vi "Virtual traverse profile.vi"(6 "N_pts":i32=100, 8 "P_end":sgl[](array[numeric])=[10.0, 0.0, 0.0], 9 "P_start":sgl[](array[numeric])=[0.0, 0.0, 0.0], 10 "U_inf":sgl[](array[numeric])=[1.0, 0.0, 0.0], 11 "Panel triangles in":T1[](array[typedef])) -> (0 "V":sgl[](array[numeric]), 1 "U":sgl[](array[numeric]), 2 "z":sgl[](array[numeric]), 3 "y":sgl[](array[numeric]), 4 "W":sgl[](array[numeric]), 5 "x":sgl[](array[numeric]))   [LabVIEW 2017]
uses:
  ctls/Triangle panel.ctl
panel:
  # "PN 26/10/17"
  # "Vertices"
  # "Edges"
  # "Unit normal"
  # "Control point"
  # "Edge\nlinks \n(tri index)"
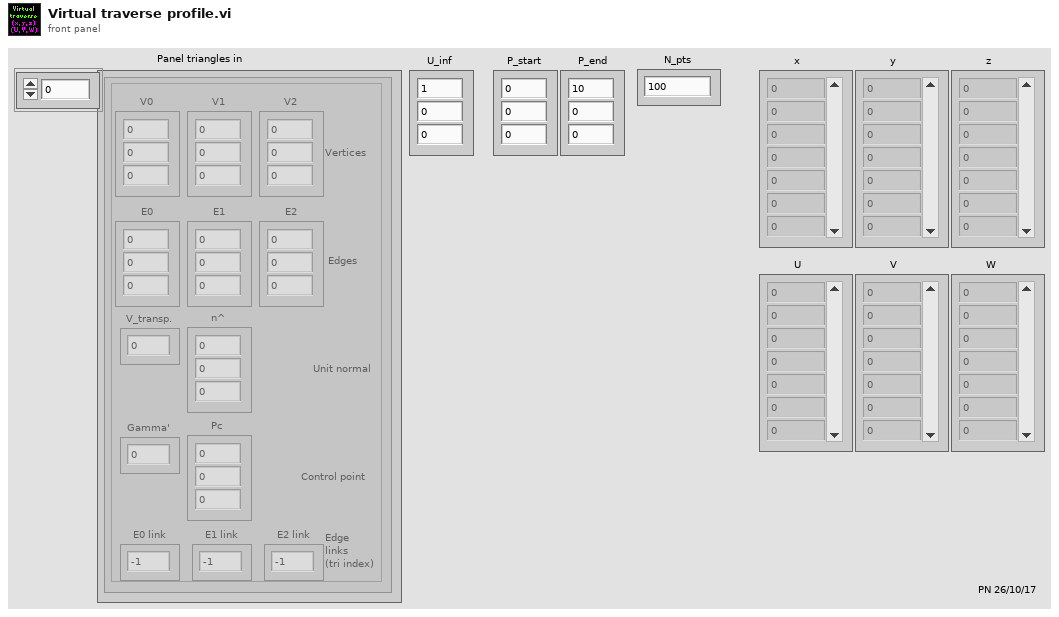
[diagram p1: front panel]
types:
  T1 = typedef "Triangle panel.ctl" = cluster{"V0":sgl[], "V1":sgl[], "V2":sgl[], "E0":sgl[], "E1":sgl[], "E2":sgl[], "n^":sgl[], "Pc":sgl[], "Gamma'":sgl, "V_transp.":sgl, "E0 link":i32, "E1 link":i32, "E2 link":i32}
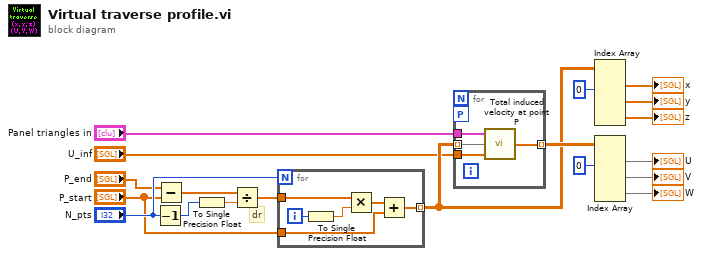
[diagram p0: block diagram]
diagram:
  # "dr"
  n1 = Decrement(x="N_pts") -> (x-1=w17:i32)
  n2 = Subtract(x="P_end", y="P_start") -> (x-y=w19:sgl[])
  n3 = To Single Precision Float(number=w17) -> (single precision float=w18:sgl)
  n4 = Divide(x=w19, y=w18) -> (x/y=w15:sgl[])
  n5 = for {
    N: "N_pts" -> [_]
    tunnel: "P_start" -> [w22]
    tunnel: w15 -> [w23]
    tunnel: [w20] -> w13 mode=indexing
    i -> [w25]
    n6 = To Single Precision Float(number=w25) -> (single precision float=w24:sgl)
    n7 = Multiply(x=w23, y=w24) -> (x*y=w21:sgl[])
    n8 = Add(x=w21, y=w22) -> (x+y=w20:sgl[])
  }
  n9 = for {
    tunnel: w13 -> [w28] mode=indexing
    tunnel: "Panel triangles in" -> [w29]
    tunnel: [w26] -> w14 mode=indexing
    tunnel: "U_inf" -> [w27]
    workers-P: _ -> [_]
    n10 = call "Total induced velocity at point P.vi"("U_inf"=w27, "P"=w28, "Triangle panels"=w29) -> ("(U, V, W) at P"=w26:sgl[])
  }
  n11 = Index Array(array=w13, index (col) #1=0 ("disabled index (col)")) -> (element #1=→"x":sgl[], element #2=→"y":sgl[], element #3=→"z":sgl[])  [unwired: 5 in]
  n12 = Index Array(array=w14, index (col) #1=0 ("disabled index (col)")) -> (element #1=→"U":sgl[], element #2=→"V":sgl[], element #3=→"W":sgl[])  [unwired: 5 in]
